vi "CleanUp.vi"(0 "object in":refnum<class "AFG3022B.lvclass">, 5 "error in (no error)":errorcluster) -> (14 "object out":refnum<class "AFG3022B.lvclass">, 19 "error out":errorcluster)   [LabVIEW 2023, in "AFG3022B.lvclass"]
uses:
  AFG3022B.lvclass
  AFG3022B.lvclass/AFG3022B.ctl
  <instrlib>/Tektronix AFG 3000 Series/Tektronix AFG 3000 Series.lvlib
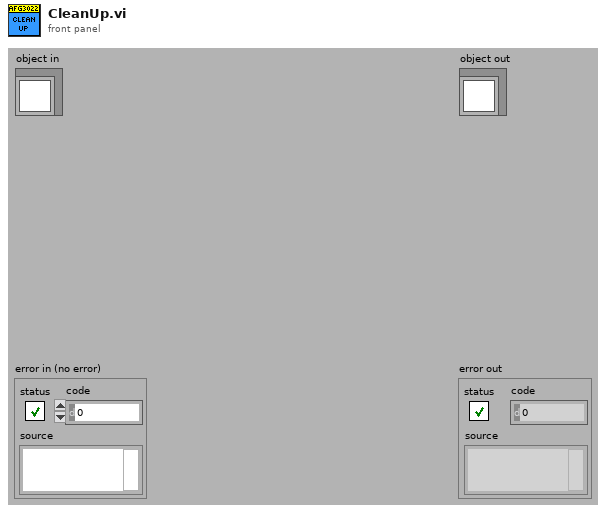
[diagram p1: front panel]
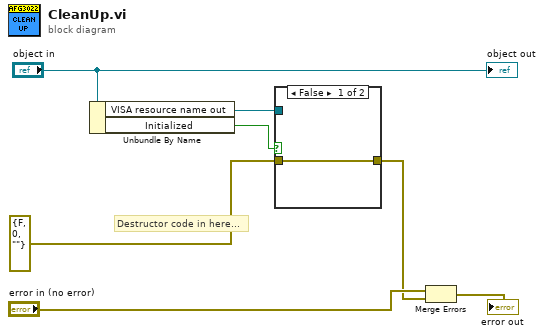
[diagram p0: block diagram]
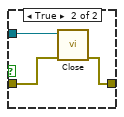
[diagram p2: hidden frame]
diagram:
  # "Destructor code in here..."
  n1 = Unbundle By Name("object in") -> ("VISA resource name out"=w3:refnum<visa-resource-name>, "Initialized"=w1:bool)
  n2 = case shown="False" w1 {
    tunnel: [w8 w11] -> w4
    tunnel: w3 -> [_ w10]
    tunnel: errorcluster {"status"=FALSE, "code"=0, "source"=""} ("error in (no error)") -> [w8 w9]
    frame False {
    }
    frame True {
      n3 = call <instrlib>:"Close.vi"("error in (no error)"=w9, "VISA resource name"=w10) -> ("error out"=w11:errorcluster)  [unwired: 9 in]
    }
  }
  n4 = Merge Errors("error in (no error)", w4) -> (→"error out":errorcluster)
  "object out" <- "object in"
